vi "Remove Discovered Object Instance by handle (incoming).vi"(10 "objectInstanceHandle":u64, 11 "hlaMap in":T1) -> (2 "deleted":bool, 3 "hlaMap out":T1)   [LabVIEW 2019, in "HLA Custom Device Engine.lvlib"]
uses:
  HLA Custom Device Engine.lvlib
  _typedefs/RThlaMapHelpers.ctl
  _typedefs/map_in_interaction.ctl
  _typedefs/map_interaction_value.ctl
  _typedefs/map_attr_param_data.ctl
  _typedefs/map_object.ctl
  _typedefs/map_object_key.ctl
  _typedefs/map_object_value.ctl
  _typedefs/map_object_instance.ctl
  _typedefs/map_object_instance_value.ctl
  _typedefs/map_object_vs_instance.ctl
  _typedefs/map_out_vs_ch_instanceId.ctl
  _typedefs/map_out_vs_ch_objects.ctl
  _typedefs/map_out_vs_ch_objects_value.ctl
  _typedefs/map_out_vs_ch_interactIonClass.ctl
  <vilib>/Utility/miscctls.llb/LVMapReplaceAction.ctl
  _Debug/VsDebugLibrary.lvlib
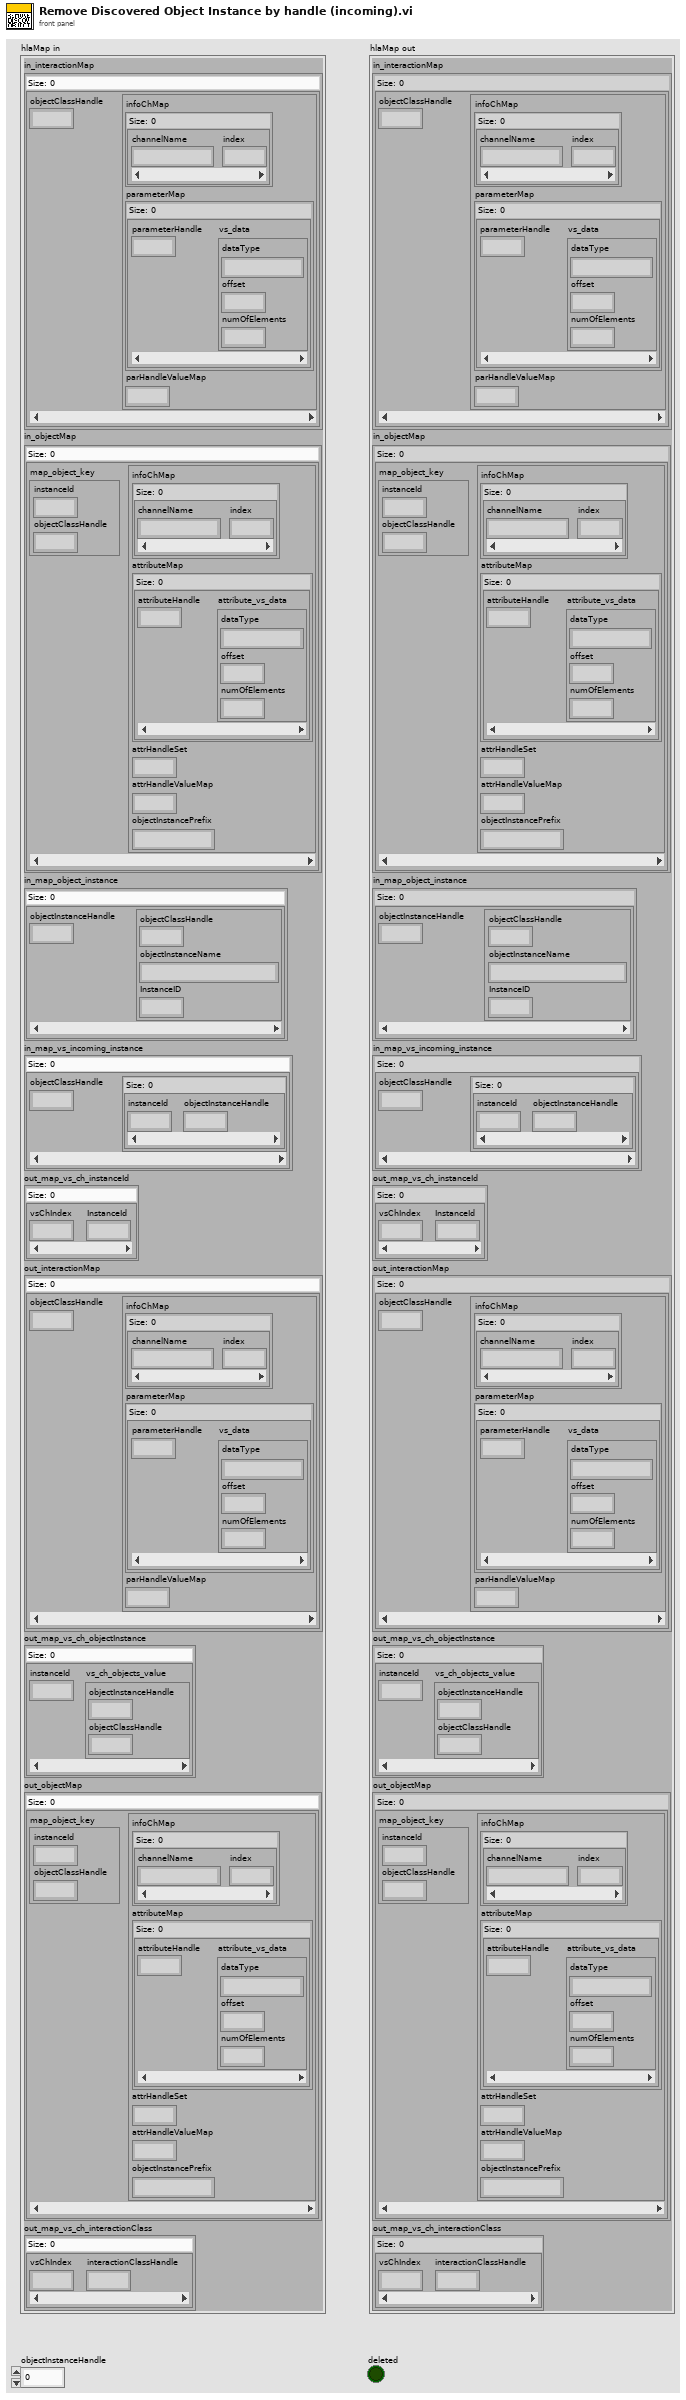
[diagram p1: front panel]
types:
  T1 = typedef "HLA Custom Device Engine.lvlib/RThlaMapHelpers.ctl" = cluster{"in_interactionMap":T2, "in_objectMap":T5, "in_map_object_instance":T8, "in_map_vs_incoming_instance":T10, "out_map_vs_ch_instanceId":T11, "out_interactionMap":T2, "out_map_vs_ch_objectInstance":T12, "out_objectMap":T5, "out_map_vs_ch_interactionClass":T14}
  T2 = typedef "HLA Custom Device Engine.lvlib/map_in_interaction.ctl" = map{u64, T3}
  T3 = typedef "HLA Custom Device Engine.lvlib/map_interaction_value.ctl" = cluster{"infoChMap":map{string, i32}, "parameterMap":map{u64, T4}, "parHandleValueMap":u64}
  T4 = typedef "HLA Custom Device Engine.lvlib/map_attr_param_data.ctl" = cluster{"dataType":string, "offset":i32, "numOfElements":i32}
  T5 = typedef "HLA Custom Device Engine.lvlib/map_object.ctl" = map{T6, T7}
  T6 = typedef "HLA Custom Device Engine.lvlib/map_object_key.ctl" = cluster{"instanceId":i32, "objectClassHandle":u64}
  T7 = typedef "HLA Custom Device Engine.lvlib/map_object_value.ctl" = cluster{"infoChMap":map{string, i32}, "attributeMap":map{u64, T4}, "attrHandleSet":u64, "attrHandleValueMap":u64, "objectInstancePrefix":string}
  T8 = typedef "HLA Custom Device Engine.lvlib/map_object_instance.ctl" = map{u64, T9}
  T9 = typedef "HLA Custom Device Engine.lvlib/map_object_instance_value.ctl" = cluster{"objectClassHandle":u64, "objectInstanceName":string, "InstanceID":i32}
  T10 = typedef "HLA Custom Device Engine.lvlib/map_object_vs_instance.ctl" = map{u64, map{i32, u64}}
  T11 = typedef "HLA Custom Device Engine.lvlib/map_out_vs_ch_instanceId.ctl" = map{i32, i32}
  T12 = typedef "HLA Custom Device Engine.lvlib/map_out_vs_ch_objects.ctl" = map{i32, T13}
  T13 = typedef "HLA Custom Device Engine.lvlib/map_out_vs_ch_objects_value.ctl" = cluster{"objectInstanceHandle":u64, "objectClassHandle":u64}
  T14 = typedef "HLA Custom Device Engine.lvlib/map_out_vs_ch_interactIonClass.ctl" = map{i32, u64}
  T15 = typedef "LVMapReplaceAction.ctl" = enum32{"Modify Entry only if found", "Add or Modify Entry", "Delete Entry"}
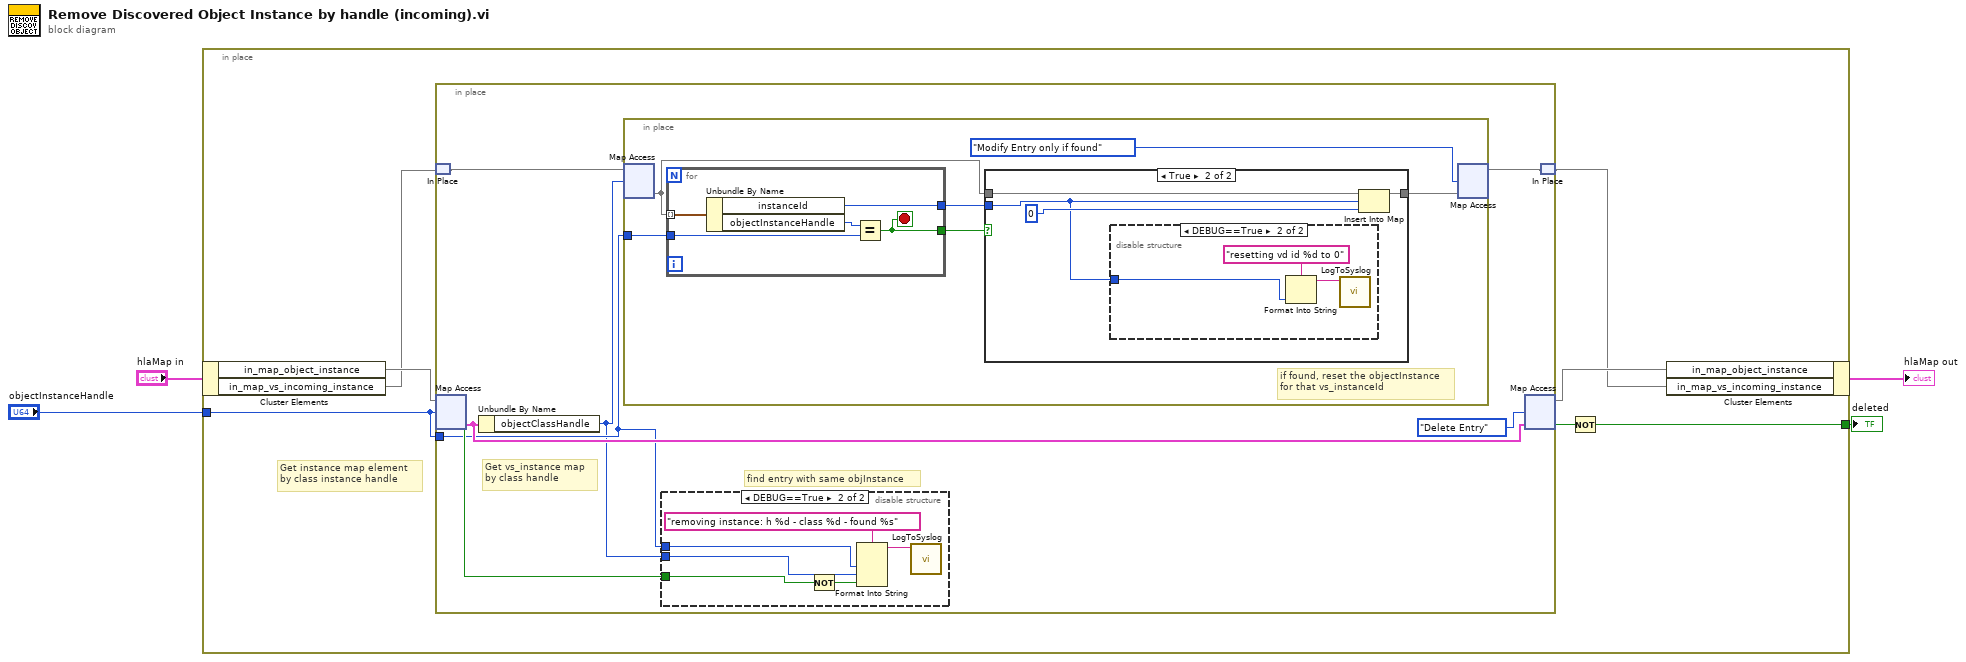
[diagram p0: block diagram]
diagram:
  n1 = in-place {
    in-place-border: "objectInstanceHandle" -> [w7]
    in-place-border: [w8] -> w1
    # "Get instance map element \nby class instance handle"
    n2 = in-place-cluster #1("hlaMap in") -> ("in_map_object_instance"=w11:T8, "in_map_vs_incoming_instance"=w6:T10)
    n3 = in-place {
      in-place-border: w7 -> [w15]
      # "find entry with same objInstance"
      # "Get vs_instance map \nby class handle"
      n4 = in-place-match #2(w6) -> (w13:T10)
      n5 = in-place-map #3(w11, w7) -> (w17:T9, w16:bool)  [unwired: 1 in]
      n6 = Unbundle By Name(w17) -> ("objectClassHandle"=w14:u64)
      n7 = in-place {
        in-place-border: w15 -> [w30]
        # "if found, reset the objectInstance\nfor that vs_instanceId"
        n8 = in-place-map #4(w13, w14) -> (w29:map{i32, u64})  [unwired: 1 in, 1 out]
        n9 = for {
          tunnel: w29 -> [w43] mode=indexing
          tunnel: w30 -> [w41]
          tunnel: [w40] -> w28
          tunnel: [w39] -> w27
          stop <- w40 stop-if-true
          n10 = Unbundle By Name(w43) -> ("instanceId"=w39:i32, "objectInstanceHandle"=w42:u64)
          n11 = Equal?(x=w42, y=w41) -> (x = y?=w40:bool)
        }
        n12 = case shown="True" w28 {
          tunnel: w29 -> [w31 w35]
          tunnel: w27 -> [_ w32]
          tunnel: [w31 w33] -> w26
          frame False {
          }
          frame True {
            n13 = disable-structure shown="DEBUG==True" {
              disable-tunnel: w32 -> [_ w38]
              frame condition #0 {
              }
              frame condition #1 (active) {
                n14 = Format Into String(format string="resetting vd id %d to 0" ("message"), w38) -> (resulting string=w36:string)  [unwired: 2 in, 1 out]
                n15 = call "LogToSyslog.vi"("message"=w36) -> ()  [unwired: 9 in, 2 out]
              }
            }
            n16 = Insert Into Map(map in=w35, key=w32, value=u64 0) -> (map out=w33:map{i32, u64})  [unwired: 2 out]
          }
        }
        n17 = in-place-map #4(w26, LVMapReplaceAction."Modify Entry only if found" ("action")) -> (w12:T10)  [unwired: 2 out]
      }
      n18 = disable-structure shown="DEBUG==True" {
        disable-tunnel: w14 -> [_ w22]
        disable-tunnel: w15 -> [_ w23]
        disable-tunnel: w16 -> [_ w24]
        frame condition #0 {
        }
        frame condition #1 (active) {
          n19 = Not(x=w24) -> (.not. x?=w19:bool)
          n20 = Format Into String(format string="removing instance: h %d - class %d - found %s" ("message"), w23, w22, w19) -> (resulting string=w20:string)  [unwired: 2 in, 1 out]
          n21 = call "LogToSyslog.vi"("message"=w20) -> ()  [unwired: 9 in, 2 out]
        }
      }
      n22 = in-place-map #3(w17, LVMapReplaceAction."Delete Entry" ("action")) -> (w10:T8, w9:bool)  [unwired: 1 out]
      n23 = in-place-match #2(w12) -> (w5:T10)
    }
    n24 = Not(x=w9) -> (.not. x?=w8:bool)
    n25 = in-place-cluster #1("in_map_object_instance"=w10, "in_map_vs_incoming_instance"=w5) -> (→"hlaMap out":T1)
  }
  "deleted" <- w1
